vi "Monitor CPU.vi"() -> ()   [LabVIEW 2013]
doc: "The Simple Task Monitor makes use of .NET assemblies to monitor basic CPU and system memory usage. It uses the PerformanceCounter class to get the CPU usage and also to determine how much memory is being used. The Process class is used to get the processes running on the system. These values are polled at 1 second intervals.\n\nThe example makes use of the System.Diagnostics.PerformanceCounter and the System.Diagnostics.Process classes.\n\nThe actual PerformanceCounter category names and counterNames were obtained from the Microsoft documentation for the PerformanceCounter class.\n\nFor more information about the various .NET libraries used in this example, please refer to the Microsoft Developers Network at msdn.microsoft.com"
panel:
  in  "update every (ms)":u32=500
  in  "stop":bool
  in  "Tab Control":enum32{"CPU Usage"}(tab)
  out "CPU Usage History":sgl(graph)
  out "CPU Usage":sgl(slide) scale=0.0..100.0
  # "Instructions:\n1. Hit the Run arrow to start the VI.\n2. Click on the appropriate tabs to display the CPU Usage History,\n     the Memory Usage History and  the list of processes.\n3. Hit Stop to stop the monitoring process.\n\nSee File>>VI Properties>>Documentation for additional information.\n\nNOTE:  This example requires Administrator privileges."
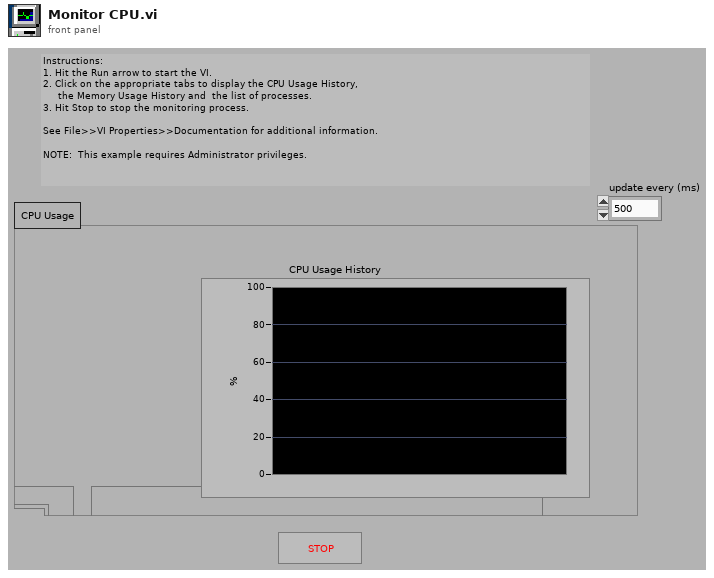
[diagram p1: front panel]
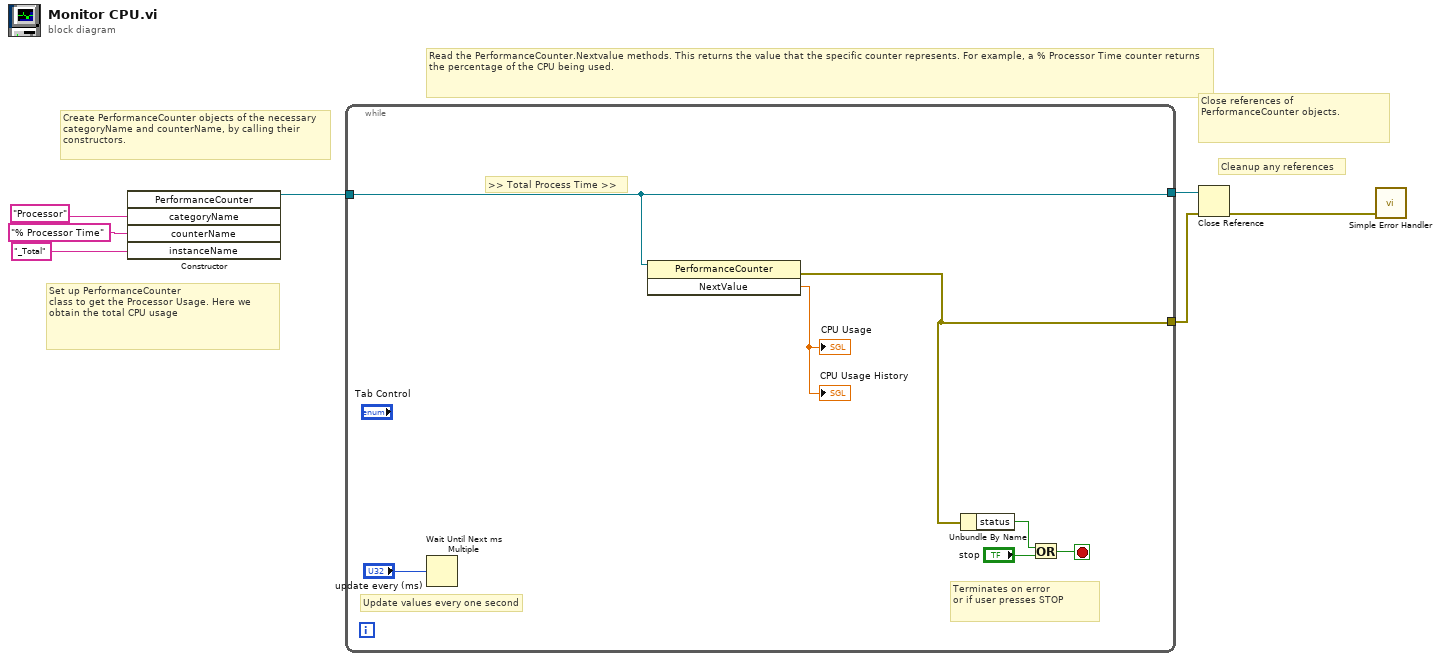
[diagram p0: block diagram]
diagram:
  # "Read the PerformanceCounter.Nextvalue methods. This returns the value that the specific counter represents. For example, a % Processor Time counter returns the percentage of the CPU being used."
  # "Close references of PerformanceCounter objects."
  # "Create PerformanceCounter objects of the necessary categoryName and counterName, by calling their constructors."
  # "Cleanup any references"
  # "Set up PerformanceCounter \nclass to get the Processor Usage. Here we obtain the total CPU usage"
  n1 = constructor class="PerformanceCounter"("categoryName"="Processor", "counterName"="% Processor Time", "instanceName"="_Total") -> (reference out=w2:refnum<k24>)  [unwired: 3 in, 5 out]
  n2 = while {
    tunnel: w2 -> [w10]
    tunnel: [w10] -> w7
    tunnel: [w9] -> w6
    stop <- w11 stop-if-true
    # ">> Total Process Time >>"
    # "Terminates on error\nor if user presses STOP"
    # "Update values every one second"
    n3 = Wait Until Next ms Multiple(millisecond multiple="update every (ms)") -> ()  [unwired: 1 out]
    n4 = invoke class="PerformanceCounter" method="NextValue"(reference=w10) -> (error out=w9:errorcluster, "NextValue"=→"CPU Usage History" →"CPU Usage":sgl)  [unwired: 2 in, 1 out]
    n5 = Unbundle By Name(w9) -> ("status"=w13:bool)
    n6 = Or(x=w13, y="stop") -> (x .or. y?=w11:bool)
  }
  n7 = Close Reference(reference=w7, error in (no error)=w6) -> (error out=w1:errorcluster)
  n8 = call <vilib>:"Simple Error Handler.vi"("error in (no error)"=w1) -> ()  [unwired: 1 in, 8 out]
